vi "Mydaq12.vi"() -> ()   [LabVIEW 2025]
panel:
  in  "steps_per_decade":dbl
  in  "stop_frequency_Hz":dbl
  in  "start_frequency_Hz":dbl
  out "Phase":T1(graph)
  out "Gain DB":T2(graph)
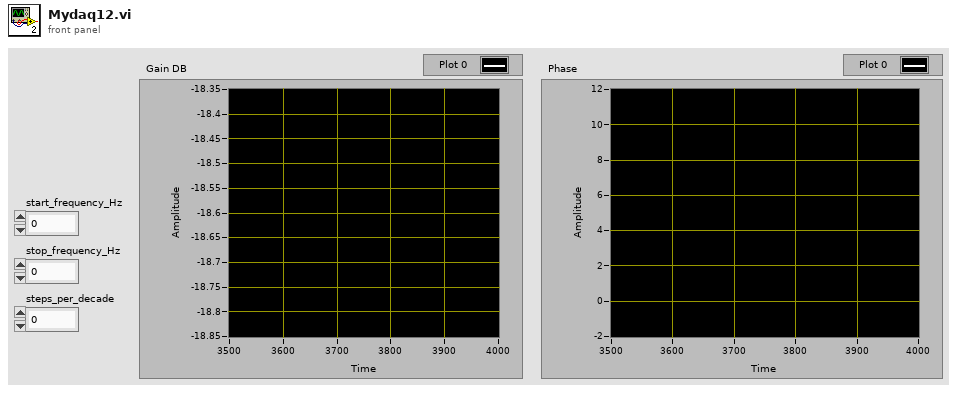
[diagram p1: front panel]
types:
  T1 = cluster{"Frequency array":dbl[], "Phase array":dbl[]}
  T2 = cluster{"Frequency array":dbl[], "Gain array":dbl[]}
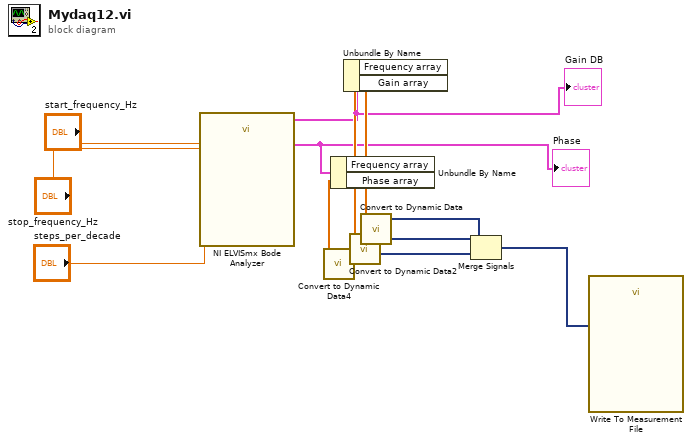
[diagram p0: block diagram]
diagram:
  n1 = call "NI ELVISmx Bode Analyzer"("Start Freq (Hz)"="start_frequency_Hz", "Stop Freq (Hz)"="stop_frequency_Hz", "Steps"="steps_per_decade") -> ("Gain Data"=w4:T2, "Phase Data"=w5:T1)  [unwired: 14 in, 1 out]
  "Gain DB" <- w4
  "Phase" <- w5
  n2 = Unbundle By Name(w5) -> ("Phase array"=w8:dbl[])  [unwired: 1 out]
  n3 = call "Convert to Dynamic Data4"("Array"=w8) -> ("Dynamic Data Type"=w11:dynamicdata)  [unwired: 3 in]
  n4 = Unbundle By Name(w4) -> ("Frequency array"=w6:dbl[], "Gain array"=w7:dbl[])
  n5 = call "Convert to Dynamic Data2"("Array"=w7) -> ("Dynamic Data Type"=w10:dynamicdata)  [unwired: 3 in]
  n6 = call "Convert to Dynamic Data"("Array"=w6) -> ("Dynamic Data Type"=w9:dynamicdata)  [unwired: 3 in]
  n7 = Merge Signals(w9, w10, w11) -> (w12:dynamicdata)
  n8 = call "Write To Measurement File"("Signals"=w12) -> ()  [unwired: 16 in, 3 out]
